vi "EnableTimer.vi"(8 "error in (no error)":errorcluster, 9 "Enable?":bool, 10 "Name":string, 11 "TimerEngine in":refnum<class "TimerEngine.lvclass">) -> (0 "error out":errorcluster, 3 "TimerEngine out":refnum<class "TimerEngine.lvclass">)   [LabVIEW 2017, in "TimerEngine.lvlib" / "TimerEngine.lvclass"]
uses:
  TimerEngine.lvclass
  TimerEngine.lvclass/TimerEngine.ctl
  _TimerClass/Timer.lvclass/Timer.ctl
  _TimerClass/Timer.lvclass
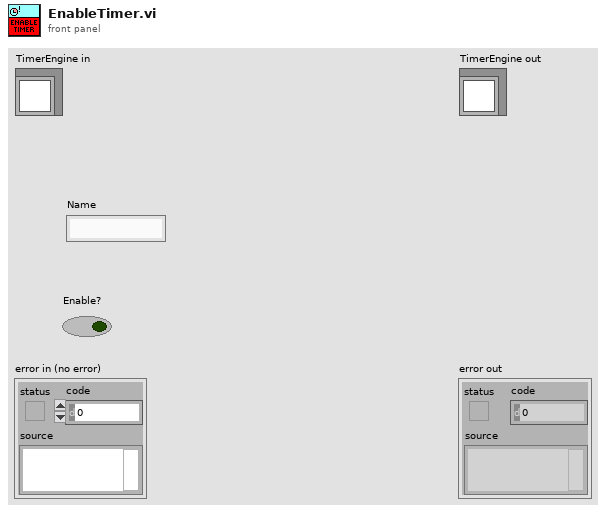
[diagram p1: front panel]
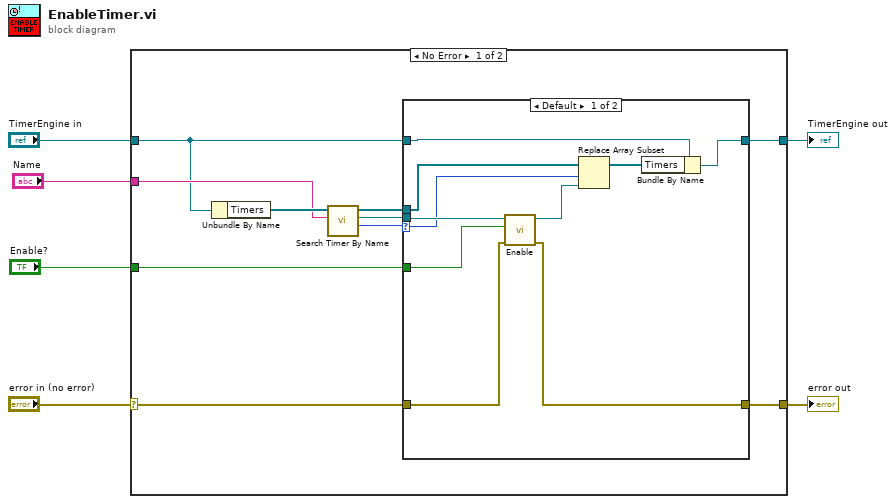
[diagram p0: block diagram]
diagram:
  n1 = case shown="No Error" "error in (no error)" {
    selector: "error in (no error)" -> [w11 w30]
    tunnel: [w10 w30] -> w5
    tunnel: [w9 w29] -> w3
    tunnel: "TimerEngine in" -> [w8 w29]
    tunnel: "Name" -> [w15 _]
    tunnel: "Enable?" -> [w13 _]
    frame No Error {
      n2 = Unbundle By Name(w8) -> ("Timers"=w16:refnum<class "Timer.lvclass">[])
      n3 = call "Search Timer By Name.vi"("Name"=w15, "Array"=w16) -> ("index of element"=w14:i32, "element"=w12:refnum<class "Timer.lvclass">, "Array 2"=w7:refnum<class "Timer.lvclass">[])  [unwired: 6 in, 1 out]
      n4 = case shown="Default" w14 {
        selector: w14 -> [w17 _]
        tunnel: w13 -> [w25 _]
        tunnel: w12 -> [w26 _]
        tunnel: w11 -> [w24 w28]
        tunnel: [w23 w28] -> w10
        tunnel: [w20 w27] -> w9
        tunnel: w8 -> [w22 w27]
        tunnel: w7 -> [w21 _]
        frame Default {
          n5 = call "Enable.vi"("error in (no error)"=w24, "Start?"=w25, "Timer in"=w26) -> ("error out"=w23:errorcluster, "Timer out"=w18:refnum<class "Timer.lvclass">)  [unwired: 7 in]
          n6 = Replace Array Subset(array=w21, new element=w18, index=w17) -> (w19:refnum<class "Timer.lvclass">[])
          n7 = Bundle By Name(cluster=w22, "Timers"=w19) -> (w20:refnum<class "TimerEngine.lvclass">)
        }
        frame -1 {
        }
      }
    }
    frame Error {
    }
  }
  "error out" <- w5
  "TimerEngine out" <- w3
